vi "Event handler-VidRec enable in funct.vi"(11 "Video Record-Funct acq.NewVal":bool) -> ()   [LabVIEW 2013]
uses:
  Typedefs/Read Write Enum.ctl
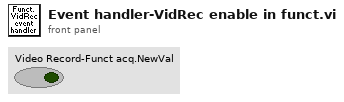
[diagram p1: front panel]
types:
  T1 = typedef "Read Write Enum.ctl" = enum16{"Read", "Write"}
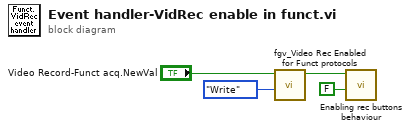
[diagram p0: block diagram]
diagram:
  n1 = call "fgv_Video Rec Enabled for Funct protocols.vi"("Function"=Read_Write_Enum."Write", "Video Recording Enabled for functional acq protocols"="Video Record-Funct acq.NewVal") -> ("Video Recording Enabled for functional acq protocols"=w4:bool)  [unwired: 9 in]
  n2 = call "Enabling rec buttons behaviour.vi"("Live img"=FALSE ("Value (Signaling)"), "New Value"=w4) -> ()  [unwired: 10 in]
